vi "ATS_Dev_Specs.vi"(0 "Device":i32, 5 "Clock":T7 {"ClckEdge" items=["Rising", "Falling"]; "ClckRate" items=["1 kS/s", "2 kS/s", "5 kS/s", "10 kS/s", "20 kS/s", "50 kS/s", "100 kS/s", "200 kS/s", "500 kS/s", "1 MS/s", "2 MS/s", "5 MS/s", "10 MS/s", "20 MS/s", "25 MS/s", "50 MS/s", "100 MS/s", "125 MS/s", "200 MS/s", "250 MS/s", "500 MS/s", "1 GS/s"]}, 7 "Input_Chan":T6 {"Range" items=["20mv", "40mV", "50mV", "80mV", "100mV", "200mV", "400mV", "500mV", "800mV", "1 V", "2 V", "4 V", "5 V", "8 V", "10 V", "20 V"]}, 12 "Update_Only":bool) -> (3 "Dev_Spec":T11, 4 "Rate_Out":cluster{"Text":string, "Rate":i32}, 6 "Range_Out":cluster{"Text":string, "Range":u32}[](array[cluster]), 8 "Output_Chan":T1[](array[typedef]) {"Range" items=["40mV", "100mV", "200mV", "400mV", "1 V", "2 V", "4 V"]}, 14 "Clock_Output":T7 {"ClckEdge" items=["Rising", "Falling"]; "ClckRate" items=["1 kS/s", "2 kS/s", "5 kS/s", "10 kS/s", "20 kS/s", "50 kS/s", "100 kS/s", "200 kS/s", "500 kS/s", "1 MS/s", "2 MS/s", "5 MS/s", "10 MS/s", "20 MS/s", "50 MS/s", "100 MS/s", "250 MS/s", "500 MS/s"]})   [LabVIEW 2010]
doc: "_____AlazarTech, Scope_____\n\nGet the Specification of the DeviceIn board.\nThe Dev_Spec indicate the name of the device and all sampling rate and input range of the device in array of text.\nThese array can be use to set the String[] in property node of a Text selector.\n\nInput:\n\"DeviceIn\" = Board to get the specification\n\"Rate_In\" = Sampling rate to select in Device specifications\n\"Range_A\" = Input range of channel A to select in Device specifications\n\"Range_B\" = Input range of channel B to select in Device specifications\n\"Update_Only\" = Read actual setting.\n\nOutput\n\"Specifications\" = specification of the board.\n\"Name\" = string of the ATS board identification\n\"Rate\" = list of available Sampling Rate in a string array format\n\n\"Rate_Out\" = sampling rate in text format and corresponding rate#.\n\"Range\" = list of available Input range in a string array format\n\"RangeA_out\" = Value in text and Range #\n\"RangeB_out\" = Value in text and Range #"
uses:
  ATS_ctl/ATS_Card_Spec.ctl
  ATS_ctl/Clock.ctl
  ATS_ctl/ClockSource.ctl
  ATS_ctl/ClockRate.ctl
  ATS_ctl/ClockEdge.ctl
  ATS_ctl/ATS_InputArray.ctl
  ATS_ctl/InputCtrl.ctl
  ATS_ctl/Coupling.ctl
  ATS_ctl/Range.ctl
  ATS_ctl/Impedance.ctl
  ATS_ctl/Bandwidth.ctl
  ATS_ctl/ATS_Global_Ctrl.ctl
panel:
  in  "Rate_In":u32
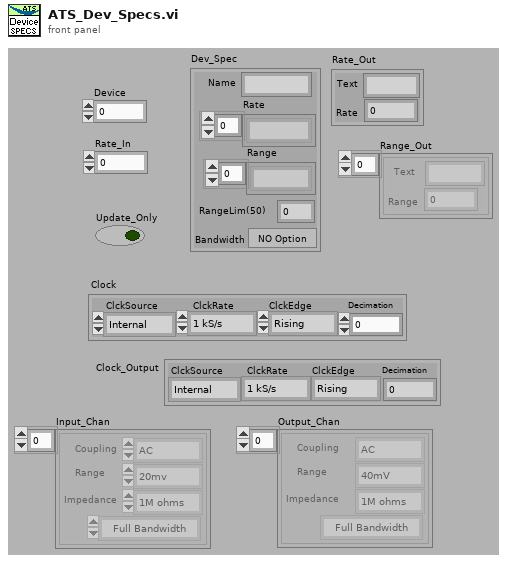
[diagram p1: front panel]
types:
  T1 = typedef "InputCtrl.ctl" = cluster{"Coupling":T2, "Range":T3, "Impedance":T4, "Bandwidth":T5}
  T2 = typedef "Coupling.ctl" = enum16{"AC", "DC"}
  T3 = typedef "Range.ctl" = u32
  T4 = typedef "Impedance.ctl" = enum16{"1M ohms", "50 ohms"}
  T5 = typedef "Bandwidth.ctl" = enum16{"Full Bandwidth", "Reduce Bandwidth"}
  T6 = typedef "ATS_InputArray.ctl" = T1[]
  T7 = typedef "Clock.ctl" = cluster{"ClckSource":T8, "ClckRate":T9, "ClckEdge":T10, "Decimation":u32}
  T8 = typedef "ClockSource.ctl" = enum16{"Internal", "External", "Medium Ext.", "Slow Ext.", "Ext. AC", "Ext. DC", "Ext. (PLL)"}
  T9 = typedef "ClockRate.ctl" = u32
  T10 = typedef "ClockEdge.ctl" = u16
  T11 = typedef "ATS_Card_Spec.ctl" = cluster{"Name":string, "Rate":string[], "Range":string[], "RangeLim(50)":u32, "Bandwidth":bool}
  T12 = typedef "ATS_Global_Ctrl.ctl" = enum16{"Init_Device", "Clear_ALL", "Set", "Get"}
  T13 = typedef "ATS_Global_4Ch.ctl" = cluster{"Record":T14, "Clock":T7, "Inputs":T6, "Trigger":T15}
  T14 = typedef "Record.ctl" = cluster{"Count":u32, "Presize":u32, "Length":u32}
  T15 = typedef "ATS_Trigger_4Ch.ctl" = cluster{"TrigOperation":T16, "Timeout (s)":dbl, "Trig. Delay":u32, "Engine X":T17, "Engine Y":T17, "ExtTrigControl":T19}
  T16 = typedef "TriggerOperation.ctl" = enum16{"Only X", "Only Y", "X or Y", "X and Y", "X xor Y", "X and not Y", "not X and Y"}
  T17 = typedef "ATS_TriggerEngine_4Ch.ctl" = cluster{"Source":T18, "Slope":enum32{"Positive", "Negative"}, "Level":u32}
  T18 = typedef "ATS_TriggerSource_4Ch.ctl" = enum32{"Chan_A", "Chan_B", "External", "Disable", "Chan_C", "Chan_D"}
  T19 = typedef "ExtTrigger.ctl" = cluster{"Coupling":T2, "Range":T20}
  T20 = typedef "ExtTrigRange.ctl" = enum16{"1 V", "5 V", "TTL"}
  T21 = typedef "Device_Info.ctl" = cluster{"Handle":u32, "Board":string, "CPLD":string, "MemorySize":u32, "SampleSize":u8, "ID":i32, "High_Memory":bool, "Chan/Board":u8}
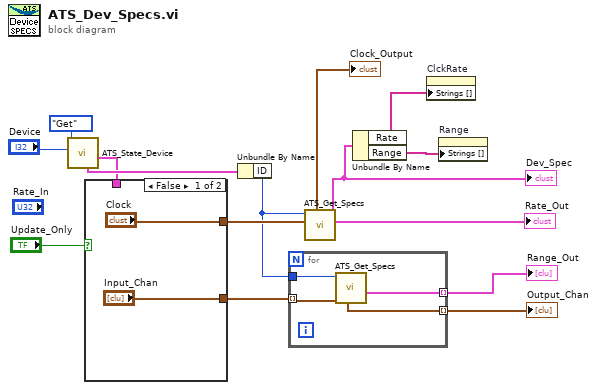
[diagram p0: block diagram]
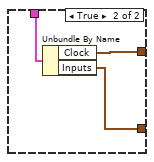
[diagram p2: hidden frame]
diagram:
  n1 = call "ATS_State_Device.vi"("DeviceIn"="Device", "ATS_GBL_Ctrl"=ATS_Global_Ctrl."Get") -> ("SetupOut"=w10:T13, "DevInfo_Out"=w13:T21)  [unwired: 4 in, 4 out]
  n2 = case shown="False" "Update_Only" {
    tunnel: ["Clock" w20] -> w15
    tunnel: w10 -> [_ w19]
    tunnel: ["Input_Chan" w18] -> w5
    frame False {
    }
    frame True {
      n3 = Unbundle By Name(w19) -> ("Clock"=w20:T7, "Inputs"=w18:T6)
    }
  }
  n4 = Unbundle By Name(w13) -> ("ID"=w4:i32)
  n5 = for {
    tunnel: w5 -> [w23] mode=indexing
    tunnel: w4 -> [w24]
    tunnel: [w22] -> w3 mode=indexing
    tunnel: [w21] -> w2 mode=indexing
    n6 = call "ATS_Get_Specs.vi"("InputControl"=w23, "ID"=w24) -> ("Range_Out"=w21:cluster{"Text":string, "Range":u32}, "OutputControl"=w22:T1)  [unwired: 5 in, 3 out]
  }
  "Output_Chan" <- w3
  "Range_Out" <- w2
  n7 = call "ATS_Get_Specs.vi"("Clock_Input"=w15, "ID"=w4) -> ("Rate_Out"=→"Rate_Out":cluster{"Text":string, "Rate":u32}, "Card_Spec"=w8:T11, "Clock_Output"=→"Clock_Output":T7)  [unwired: 5 in, 2 out]
  "Dev_Spec" <- w8
  n8 = Unbundle By Name(w8) -> ("Rate"=w6:string[], "Range"=w1:string[])
  n9 = property on="ClckRate" class="Ring (strict)"("Strings []"=w6) -> ()  [unwired: 2 in, 2 out]
  n10 = property on="Range" class="Ring (strict)"("Strings []"=w1) -> ()  [unwired: 2 in, 2 out]
